vi "TalonFX_SetSensorPosition.vi"(6 "timeoutSeconds":dbl=0.05, 8 "error in (no error)":errorcluster, 10 "SetPosition":dbl, 11 "DeviceReference":T1) -> (0 "error out":errorcluster)   [LabVIEW 2023]
uses:
  <vilib>/Rock Robotics/WPI/ThirdParty/Phoenix6/DeviceReference.ctl
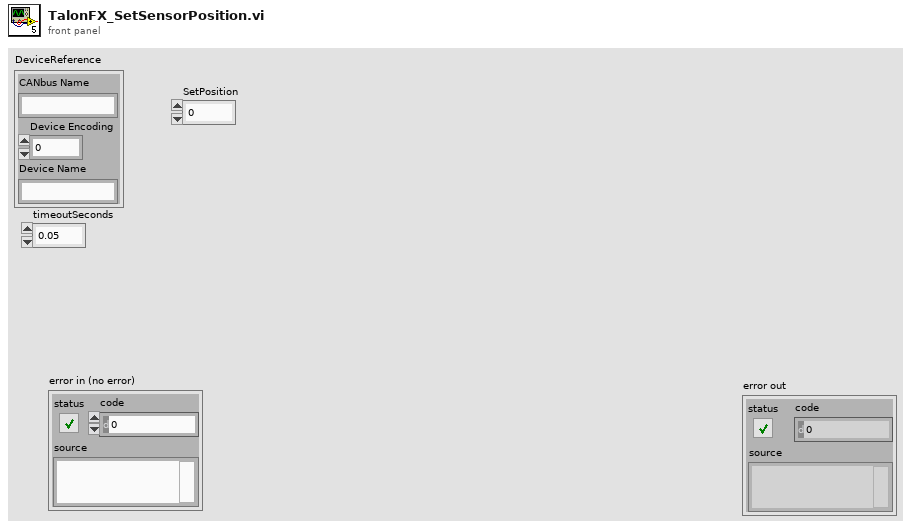
[diagram p1: front panel]
types:
  T1 = typedef "DeviceReference.ctl" = cluster{"CANbus Name":string, "Device Encoding":u32, "Device Name":string}
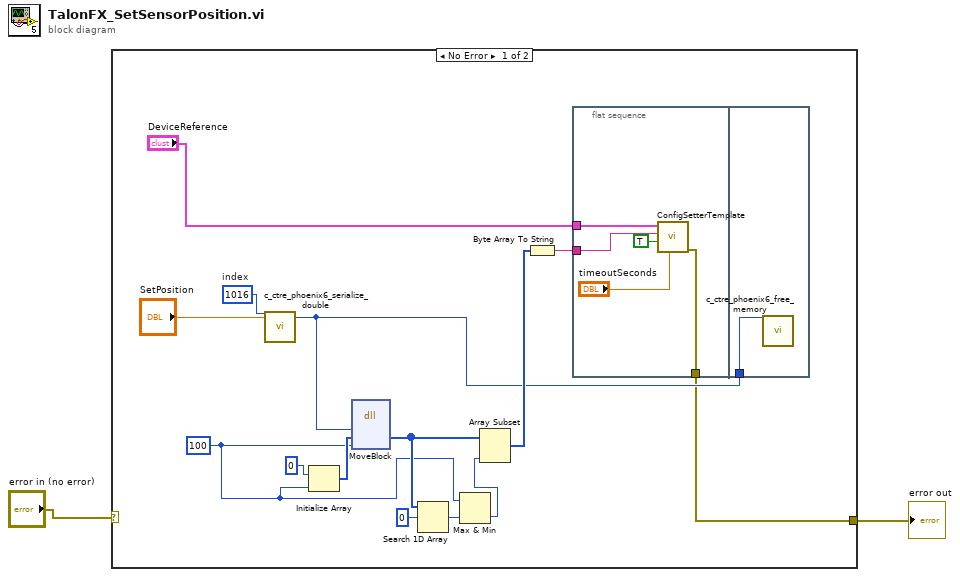
[diagram p0: block diagram]
diagram:
  n1 = case shown="No Error" "error in (no error)" {
    selector: "error in (no error)" -> [_ w23]
    tunnel: [w3 w23] -> w1
    frame No Error {
      w10 = 1016  # index
      w5 = i64 100 ("size")
      n2 = call <vilib>:"c_ctre_phoenix6_serialize_double.vi"("Numeric 2"=w10, "Numeric 3"="SetPosition") -> ("Numeric 4"=w9:u32)  [unwired: 24 in, 1 out]
      n3 = Initialize Array(u8 0 ("element"), w5) -> (w16:u8[])
      n4 = dll-call lib="LabVIEW" fn="MoveBlock"("ps"=w9, "pd"=w16, "size"=w5) -> ("pd"=w8:u8[])  [unwired: 6 in, 2 out]
      n5 = Search 1D Array(1D array=w8, element=u8 0) -> (index of element=w6:i32)  [unwired: 1 in]
      n6 = Max & Min(x=w5, y=w6) -> (min(x,y)=w4:i64)  [unwired: 1 out]
      n7 = Array Subset(array=w8, length=w4) -> (w14:u8[])  [unwired: 1 in]
      n8 = Byte Array To String(unsigned byte array=w14) -> (string=w12:string)
      n9 = flat-sequence {
        tunnel: w12 -> [w20]
        tunnel: "DeviceReference" -> [w21]
        tunnel: [w17] -> w3
        tunnel: w9 -> [w22]
        frame #0 {
          n10 = call <vilib>:"ConfigSetterTemplate.vi"("timeoutSeconds"="timeoutSeconds", "FutureProofConfigs"=TRUE, "Configs"=w20, "DeviceReference"=w21) -> ("error out"=w17:errorcluster)  [unwired: 7 in]
        }
        frame #1 {
          n11 = call <vilib>:"c_ctre_phoenix6_free_memory.vi"("Numeric 3"=w22) -> ()  [unwired: 25 in, 2 out]
        }
      }
    }
    frame Error {
    }
  }
  "error out" <- w1
